vi "ItemNames Write.vi"(4 "error in (no error)":errorcluster, 5 "Value":string[](array[string]), 6 "Container State":T2, 7 "Display State In":T1) -> (0 "error out":errorcluster, 3 "Display State Out":T1)   [LabVIEW 2014, in "ListBox XControl.xctl"]
uses:
  ListBox XControl.xctl
  <vilib>/_xctls/Container State.ctl
  State ListBox.ctl
  <vilib>/_xctls/XControlSupport.lvlib
panel:
  # "Replace the Value Control below with a Control of desired type.\nDo not remove this Control or the others from the connector pane.\nDo not change the connector pane pattern.\nThe Value control should always be the third terminal from top on the input side in the connector pane."
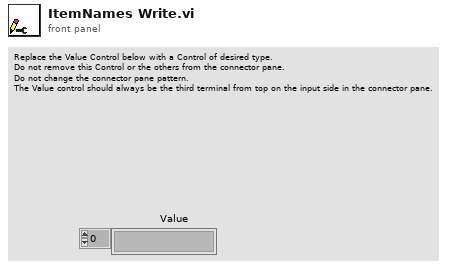
[diagram p1: front panel]
types:
  T1 = typedef "ListBox XControl.xctl/State ListBox.ctl" = cluster{"ItemNames[]":string[], "Listbox Ref":refnum<vi>, "Select All By Default":bool}
  T2 = typedef "XControlSupport.lvlib/Container State.ctl" = cluster{"Indicator?":bool, "Run Mode?":bool, " Refnum":refnum<vi>}
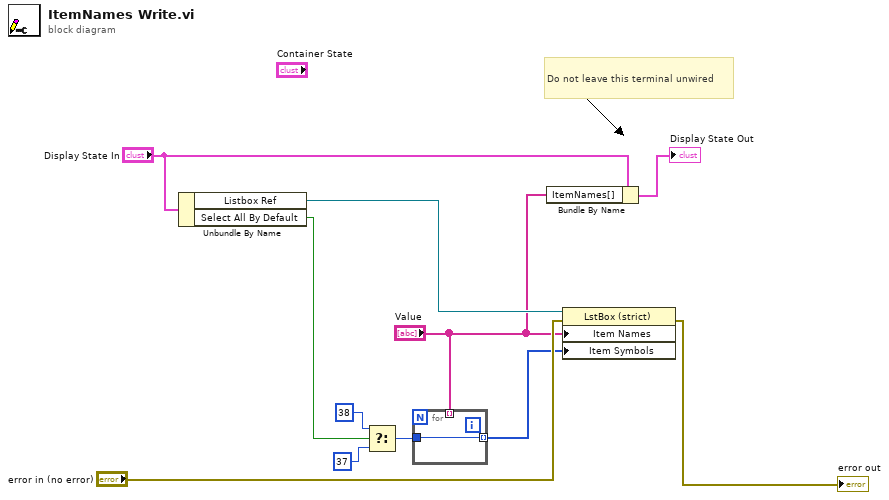
[diagram p0: block diagram]
diagram:
  # "Do not leave this terminal unwired"
  n1 = Unbundle By Name("Display State In") -> ("Listbox Ref"=w11:refnum<vi>, "Select All By Default"=w5:bool)
  n2 = Select(t=38, s=w5, f=37) -> (s? t:f=w6:i32)
  n3 = for {
    tunnel: [w12] -> w3 mode=indexing
    tunnel: w6 -> [w12]
    tunnel: "Value" -> [_] mode=indexing
  }
  n4 = Bundle By Name(cluster="Display State In", "ItemNames[]"="Value") -> (→"Display State Out":T1)
  n5 = property class="LstBox (strict)"(reference=w11, error in="error in (no error)", "Item Names"="Value", "Item Symbols"=w3) -> (error out=→"error out":errorcluster)  [unwired: 1 out]
